vi "LIA Test Frequency Shift FPGA.vi"() -> ()   [LabVIEW 2017]
uses:
  <instrlib>/_niInstr/Streaming/v1/Common/Stream State.ctl
  <vilib>/Platform/TimedLoop/XDataNode/timing_clust.ctl
  <vilib>/Platform/TimedLoop/XDataNode/nitl_modes.ctl
  <vilib>/Platform/TimedLoop/XDataNode/wakeup.ctl
  <instrlib>/_niInstr/DSP/v1/Shared/Public/IQ Data.ctl
  <vilib>/rvi/Emulation/niFpgaSctlEmulationGetInTimedLoop.vi
  <vilib>/rvi/Emulation/niFpgaEmulationReportErrorSimple.vi
  <vilib>/rvi/Emulation/niFpgaGetClockAttributes.vi
  <vilib>/rvi/Emulation/niFpgaCriticalErrorInLSC.vi
  <instrlib>/_niInstr/Basic Elements/v1/FPGA/Private/Count Up U64.vi
  <vilib>/rvi/interface/RandomDataEmulation/niFpgaRandomDataHandleErrors.vi
  <vilib>/Platform/TimedLoop/XDataNode/XDataNode.xnode
  <vilib>/rvi/DataTransferAndStorage/Container/XNode/niFpgaContainer.xnode
  <vilib>/rvi/interface/RandomDataEmulation/nirviRandomDataFpgaReadWriteTemplate.vi
  <vilib>/Platform/TimedLoop/XDataNode/XDNodeRunTimeDep.lvlib
  <instrlib>/_niInstr/DSP/v1/FPGA/niInstr DSP v1 FPGA.lvlib
  <instrlib>/_niInstr/DSP/v1/Shared/niInstr DSP v1 Shared.lvlib
  <instrlib>/_niInstr/Streaming/v1/FPGA/niInstr Streaming v1 FPGA.lvlib
  <instrlib>/_niInstr/Basic Elements/v1/FPGA/niInstr Basic Elements v1 FPGA.lvlib
  <instrlib>/_niInstr/Streaming/v1/Common/niInstr Streaming v1 Common.lvlib
panel:
  in  "output sample rate 0":fxp<+,48,1>=1.0
  in  "fractional decimator 0 (F)":bool
  out "stream control rdi count":u64
  in  "strem.force error 0":bool caption="force error (false)"
  out "FIFO rdi count":u64
  out "frequency shift rdi count":u64
  out "stream.metadata 0":u64
  out "stream.samples transferred 0":u64
  out "stream.state 0":T1
  in  "stream.request state 0":T1
  in  "stream.num samples 0":u64
  in  "nco enable (T) 0":bool=TRUE
  in  "nco frequency 0":fxp<+/-,48,0>
  in  "reset (T) 0":bool=TRUE
  in  "frequency shift 0":fxp<+/-,48,0> format="%#.48g"
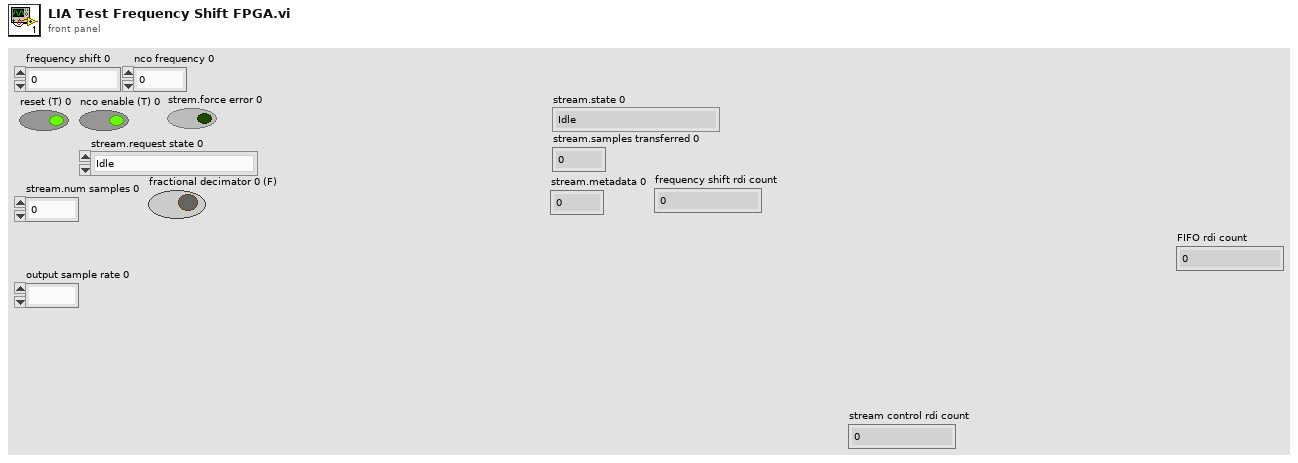
[diagram p1: front panel]
types:
  T1 = typedef "niInstr Streaming v1 Common.lvlib/Stream State.ctl" = enum8{"Idle", "Finite Transfer", "Continuous", "Done", "Error", "Not Ready", "Cancel"}
  T2 = typedef "XDNodeRunTimeDep.lvlib/timing_clust.ctl" = cluster{"Expected End [f-1]":u64, "Actual End [f-1]":u64, "Finished Late? [f-1]":bool, "Expected End [i-1]":u64, "Actual End [i-1]":u64, "Finished Late? [i-1]":bool, "Expected Start [i]":u64, "Actual Start [i]":u64, "Expected Start [f]":u64, "Actual Start [f]":u64, "Source Name":string, "Structure Name":string, "Period":i64, "Deadline":i64, "Offset":i64, "Start":i64, "Priority":i32, "Timeout":i32, "Mode":T3, "Wakeup Reason":T4, "Error":errorcluster, "Source Type":string, "Secondary Source Type":string, "Global End Time":u64, "Global Start Time":u64, "Frame Duration":u64, "Iteration Duration":u64, "Assigned CPU":i32, "I/O Scan Engine Mode":u32}
  T3 = typedef "XDNodeRunTimeDep.lvlib/nitl_modes.ctl" = enum32{"No Change", "Process missed periods, maintain original phase", "Discard missed periods, maintain original phase", "Process missed periods, ignore original phase", "Discard missed periods, ignore original phase"}
  T4 = typedef "XDNodeRunTimeDep.lvlib/wakeup.ctl" = enum32{"Normal", "Aborted", "Asynchronous wakeup", "Timing source error", "Timed loop error", "Timeout"}
  T5 = typedef "niInstr DSP v1 Shared.lvlib/IQ Data.ctl" = cluster{"I":fxp<+/-,18,1>, "Q":fxp<+/-,18,1>, "overflow":bool}
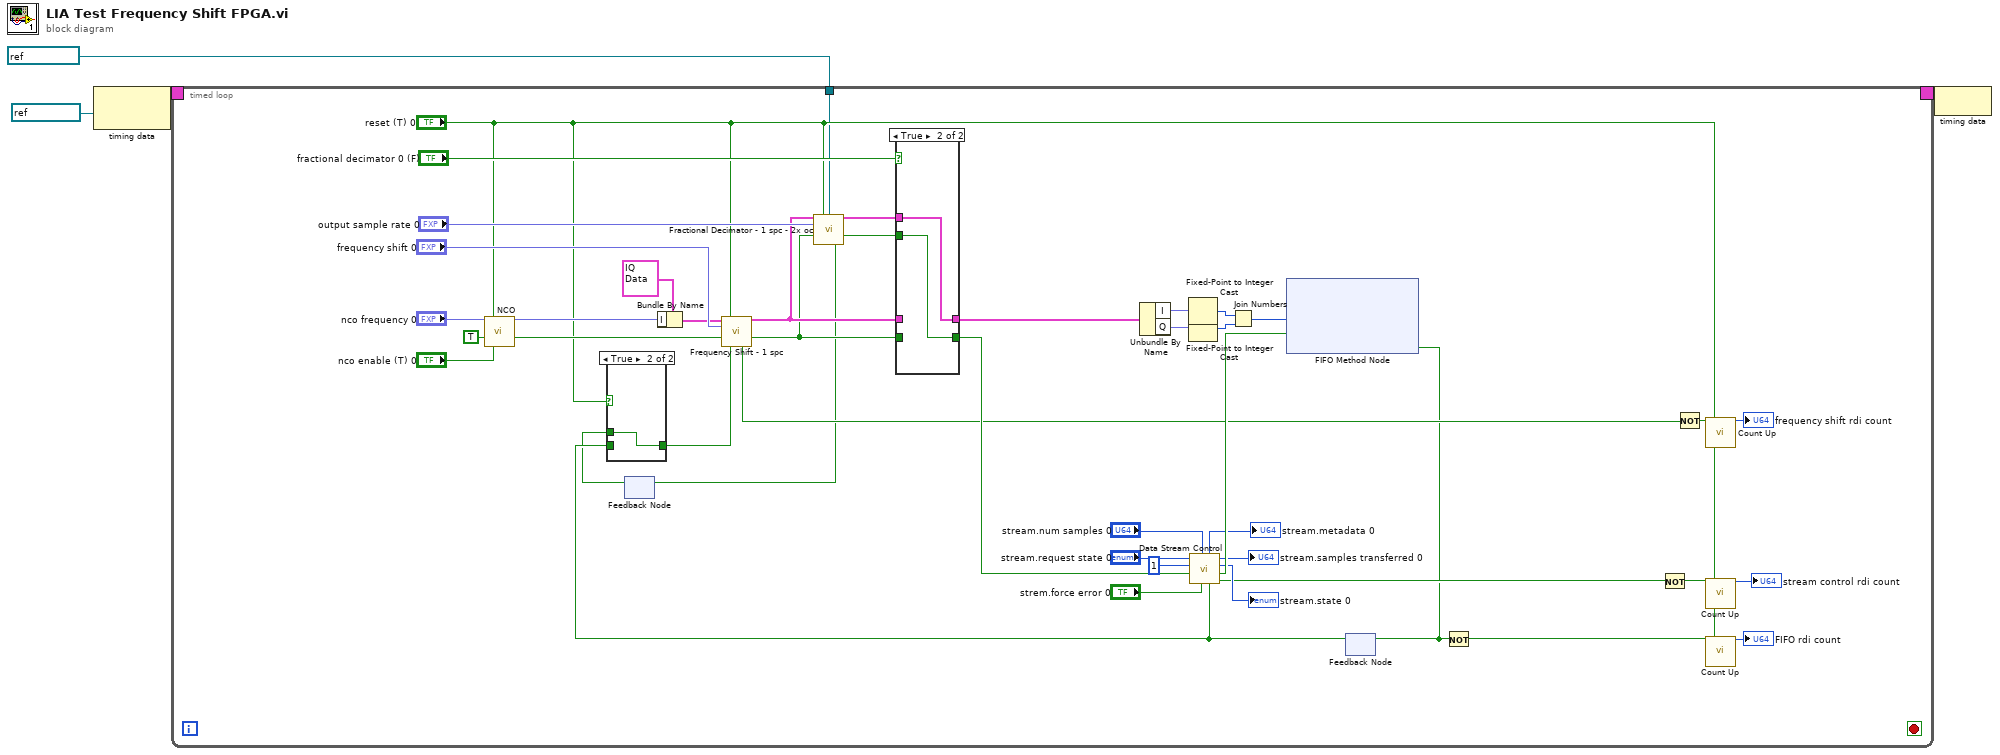
[diagram p0: block diagram]
diagram:
  n1 = node-c288(refnum<k21> "100MHz" ("Source Name")) -> (w4:T2)
  n2 = timed-loop {
    timing: w4 -> [_]
    timing-out: [_] -> w3
    tunnel: refnum<k21> "200 MHz" ("clock x 2") -> [w5]
    stop <- _ stop-if-true
    n3 = call <instrlib>:"NCO.vi"("frequency"="nco frequency 0", "reset"="reset (T) 0", "input valid"=TRUE, "enable (T)"="nco enable (T) 0") -> ("cosine out"=w45:fxp<+/-,18,1>, "output valid"=w43:bool)  [unwired: 9 in, 1 out]
    n4 = feedback #1() -> (w7:bool)  [unwired: 1 in]
    n5 = Bundle By Name(cluster=T5 {"I"=0.0, "Q"=0.0, "overflow"=FALSE} ("data in"), "I"=w45) -> (w44:T5)
    n6 = feedback #2() -> (w9:bool)  [unwired: 1 in]
    n7 = case shown="True" "reset (T) 0" {
      tunnel: w9 -> [w49 _]
      tunnel: w7 -> [_ w50]
      tunnel: [w49 w50] -> w6
      frame False {
      }
      frame True {
      }
    }
    n8 = call <instrlib>:"Frequency Shift - 1 spc.vi"("data in"=w44, "reset"="reset (T) 0", "frequency shift"="frequency shift 0", "input valid"=w43, "ready for output (T)"=w6) -> ("data out"=w16:T5, "output valid"=w14:bool, "ready for input"=w12:bool)  [unwired: 8 in]
    n9 = call <instrlib>:"Fractional Decimator - 1 spc - 2x oc.vi"("data in"=w16, "reset"="reset (T) 0", "clock x 2"=w5, "output sample rate"="output sample rate 0", "input valid"=w14) -> ("data out"=w19:T5, "output valid"=w18:bool, "ready for input"=w8:bool)  [unwired: 8 in]
    n10 = feedback-in #1(w8) -> ()
    n11 = case shown="True" "fractional decimator 0 (F)" {
      tunnel: w19 -> [_ w54]
      tunnel: w18 -> [_ w53]
      tunnel: w16 -> [w52 _]
      tunnel: [w52 w54] -> w15
      tunnel: w14 -> [w51 _]
      tunnel: [w51 w53] -> w13
      frame False {
      }
      frame True {
      }
    }
    n12 = Unbundle By Name(w15) -> ("I"=w40:fxp<+/-,18,1>, "Q"=w39:fxp<+/-,18,1>)
    n13 = Fixed-Point to Integer Cast(1:w40) -> (0:w38:i32)
    n14 = Fixed-Point to Integer Cast(1:w39) -> (0:w37:i32)
    n15 = call <instrlib>:"Data Stream Control.vi"("ready for input?"=w9, "force error"="strem.force error 0", "stream.num samples 0"="stream.num samples 0", "data valid"=w13, "element count"=u16 1, "stream.request state 0"="stream.request state 0") -> ("request data"=w22:bool, "send data"=w34:bool, "stream.state 0"=→"stream.state 0":T1, "stream.samples transferred 0"=→"stream.samples transferred 0":u64, "stream.metadata 0"=→"stream.metadata 0":u64)  [unwired: 1 in]
    n16 = Join Numbers(hi=w38, lo=w37) -> ((hi.lo)=w36:u64)
    n17 = xnode ("FIFO Method Node")("Element"=w36, "Input Valid"=w34) -> ("Ready for Input"=w11:bool)  [unwired: 1 in, 1 out]
    n18 = feedback-in #2(w11) -> ()
    n19 = Not(x=w11) -> (.not. x?=w25:bool)
    n20 = Not(x=w22) -> (.not. x?=w21:bool)
    n21 = Not(x=w12) -> (.not. x?=w28:bool)
    n22 = call-poly <instrlib>:"Count Up.vi"("increment"=w28, "reset"="reset (T) 0") -> ("count out"=→"frequency shift rdi count":u64)  [unwired: 13 in]
    n23 = call-poly <instrlib>:"Count Up.vi"("increment"=w21, "reset"="reset (T) 0") -> ("count out"=→"stream control rdi count":u64)  [unwired: 13 in]
    n24 = call-poly <instrlib>:"Count Up.vi"("increment"=w25, "reset"="reset (T) 0") -> ("count out"=→"FIFO rdi count":u64)  [unwired: 13 in]
  }
  n25 = node-c288(w3) -> ()
